vi "Set Node-ID.vi"(8 "error in":errorcluster, 10 "Node-ID":u8, 11 "CANopen Master in":refnum<class "CANopen Master.lvclass">) -> (0 "error out":errorcluster, 3 "CANopen Master out":refnum<class "CANopen Master.lvclass">)   [LabVIEW 2024, in "CANopen Master.lvlib" / "CANopen Master.lvclass"]
uses:
  CANopen Master.lvclass
  CANopen Master.lvclass/CANopen Master.ctl
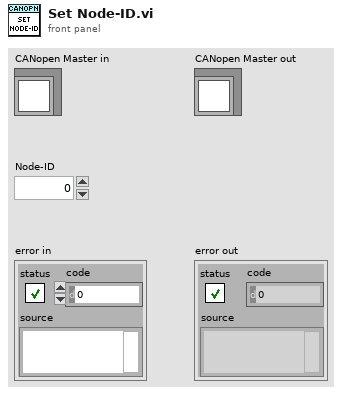
[diagram p1: front panel]
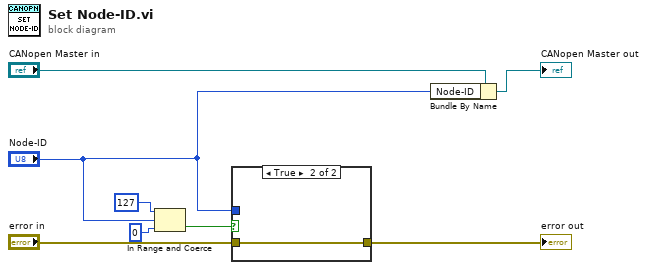
[diagram p0: block diagram]
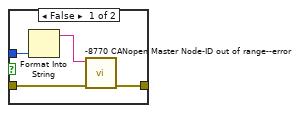
[diagram p2: hidden frame]
diagram:
  n1 = In Range and Coerce(upper limit=u8 127, x="Node-ID", lower limit=u8 0) -> (In Range?=w4:bool)  [unwired: 1 out]
  n2 = case shown="True" w4 {
    tunnel: "error in" -> [w12 w13]
    tunnel: [w11 w13] -> w8
    tunnel: "Node-ID" -> [w10 _]
    frame False {
      n3 = Format Into String(w10) -> (resulting string=w9:string)  [unwired: 3 in, 1 out]
      n4 = call "-8770 CANopen Master Node-ID out of range--error.vi"("error in"=w12, "Argument"=w9) -> ("error out"=w11:errorcluster)  [unwired: 9 in]
    }
    frame True {
    }
  }
  "error out" <- w8
  n5 = Bundle By Name(cluster="CANopen Master in", "Node-ID"="Node-ID") -> (→"CANopen Master out":refnum<class "CANopen Master.lvclass">)
